vi "Build Path.vi"(0 "Status输入":T1, 2 "VI输入":refnum<vi>, 5 "错误输入（无错误）":errorcluster) -> (14 "Status输出":T1, 19 "错误输出":errorcluster)   [LabVIEW 2013]
uses:
  Status.ctl
  Step.ctl
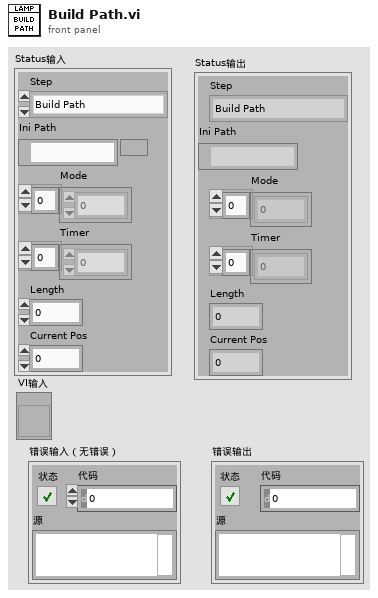
[diagram p1: front panel]
types:
  T1 = typedef "Status.ctl" = cluster{"Step":T2, "Ini Path":path, "Mode":u32[], "Timer":dbl[], "Length":i32, "Current Pos":i32}
  T2 = typedef "Step.ctl" = enum16{"Build Path", "Read Ini", "Run"}
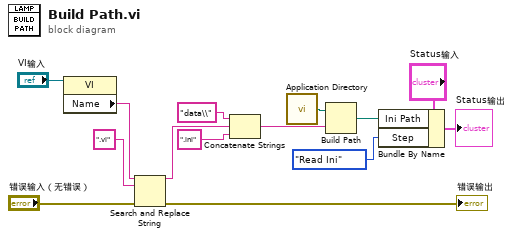
[diagram p0: block diagram]
diagram:
  n1 = property class="VI"(reference="VI输入") -> ("Name"=w11:string)  [unwired: 1 in, 2 out]
  n2 = Search and Replace String(input string=w11, search string=".vi" ("搜索字符串"), error in="错误输入（无错误）") -> (result string=w9:string, error out=→"错误输出":errorcluster)  [unwired: 5 in, 2 out]
  n3 = Concatenate Strings("data\\" ("字符串"), w9, ".ini" ("字符串")) -> (w5:string)
  n4 = call <vilib>:"Application Directory.vi"() -> ("Application Directory"=w6:path)
  n5 = Build Path(base path=w6, name or relative path=w5) -> (appended path=w2:path)
  n6 = Bundle By Name(cluster="Status输入", "Ini Path"=w2, "Step"=Step."Read Ini") -> (→"Status输出":T1)
